vi "Get_Indicies_for_Bad_Tracks_(101-11)-1.vi"(3 "[IN] Current index":i32=1, 4 "[IN] Indicies of subtracks for \ntransformation (resolving)":i32[](array[numeric]), 5 "[IN] Competed elonga\ntion is reconstructed?":bool) -> (0 "[OUT] Column Number":i32, 1 "[OUT] Row Number":i32, 2 "[OUT] Competed elonga\ntion is reconstructed?":bool)   [LabVIEW 2013]
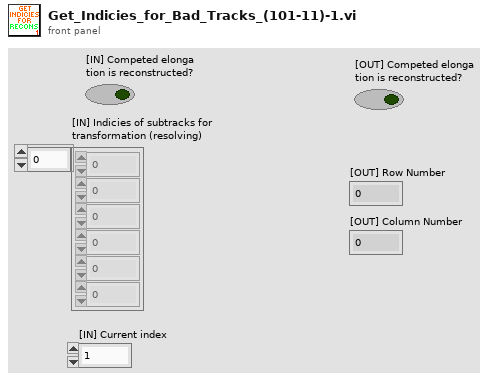
[diagram p1: front panel]
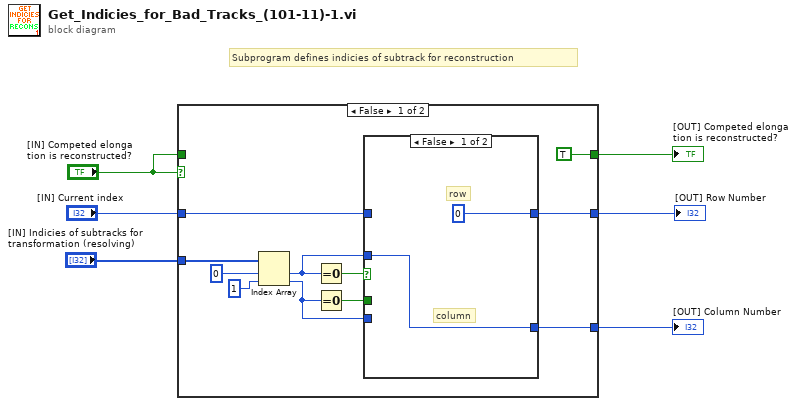
[diagram p0: block diagram]
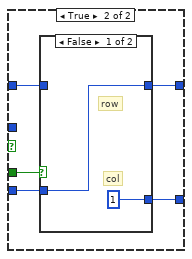
[diagram p2: hidden frame]
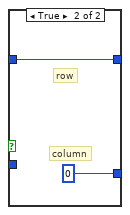
[diagram p3: hidden frame]
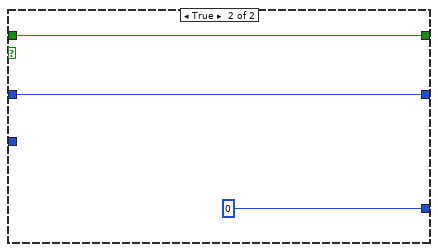
[diagram p4: hidden frame]
diagram:
  # "Subprogram defines indicies of subtrack for reconstruction"
  n1 = case shown="False" "[IN] Competed elonga\ntion is reconstructed?" {
    tunnel: "[IN] Indicies of subtracks for \ntransformation (resolving)" -> [w17 _]
    tunnel: "[IN] Current index" -> [w12 w30]
    tunnel: [w9 w30] -> w2
    tunnel: [w8 0 ("index")] -> w1
    tunnel: [TRUE w31] -> w4
    tunnel: "[IN] Competed elonga\ntion is reconstructed?" -> [_ w31]
    frame False {
      n2 = Index Array(array=w17, index #1=0 ("index"), index #2=1 ("index")) -> (element #1=w10:i32, element #2=w11:i32)
      n3 = Equal To 0?(x=w10) -> (x = 0?=w14:bool)
      n4 = Equal To 0?(x=w11) -> (x = 0?=w13:bool)
      n5 = case shown="False" w14 {
        tunnel: w13 -> [_ w24]
        tunnel: w12 -> [_ w23]
        tunnel: [0 ("[IN] Current index") w22] -> w9
        tunnel: [w18 w21] -> w8
        tunnel: w11 -> [_ w20]
        tunnel: w10 -> [w18 _]
        frame False {
          # "column"
          # "row"
        }
        frame True {
          n6 = case shown="False" w24 {
            tunnel: w23 -> [_ w28]
            tunnel: [w26 w28] -> w22
            tunnel: [1 0] -> w21
            tunnel: w20 -> [w26 _]
            frame False {
              # "col"
              # "row"
            }
            frame True {
              # "column"
              # "row"
            }
          }
        }
      }
    }
    frame True {
    }
  }
  "[OUT] Competed elonga\ntion is reconstructed?" <- w4
  "[OUT] Row Number" <- w2
  "[OUT] Column Number" <- w1
